vi "Tell Child.vi"(4 "Priority":bool, 6 "UID":string, 7 "Actor in":refnum<class "Actor.lvclass">, 8 "Error in":errorcluster, 9 "Error":errorcluster, 10 "Actor":refnum<class "Actor.lvclass">) -> (0 "Error out":errorcluster, 5 "Actor out":refnum<class "Actor.lvclass">)   [LabVIEW 2020, in "jettl.lvlib" / "Stopped jettl Msg.lvlib" / "Stopped.lvlib"]
uses:
  Stopped.lvlib
  jettl.lvlib
  Init Msg.vi
  Actor/Actor.lvclass
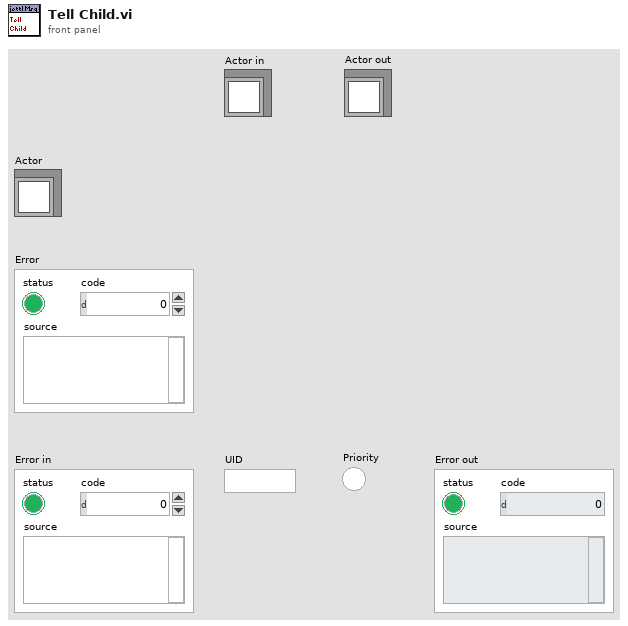
[diagram p1: front panel]
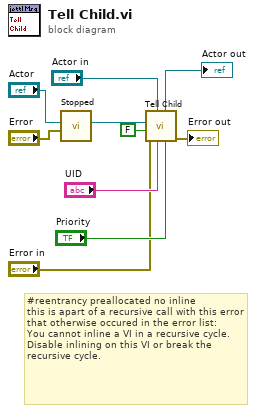
[diagram p0: block diagram]
diagram:
  # "#reentrancy preallocated no inline\nthis is apart of a recursive call with this error that otherwise occured in the error list:\nYou cannot inline a VI in a recursive cycle. Disable inlining on this VI or break the recursive cycle."
  n1 = call-poly "Stopped.vi"("Error"="Error", "Actor"="Actor") -> ("Msg"=w4:refnum<class "Msg.lvclass">)  [unwired: 9 in]
  n2 = call "Tell Child.vi"("Priority"="Priority", "UID"="UID", "Actor in"="Actor in", "Error in"="Error in", "Reply"=FALSE, "Msg"=w4) -> ("Error out"=→"Error out":errorcluster, "Actor out"=→"Actor out":refnum<class "Actor.lvclass">)  [unwired: 4 in]
